vi "ReleaseAllQueues.vi"(8 "error in (no error)":errorcluster, 11 "Message Queues":T1) -> (0 "error out":errorcluster)   [LabVIEW 2018]
uses:
  Message Queue/All Message Queues.ctl
  Message Queue/Message Cluster.ctl
  Controls/Data Queue.ctl
  Controls/Acquired Data.ctl
  Controls/Data Notifier.ctl
  Message Queue/Message Queue.lvlib
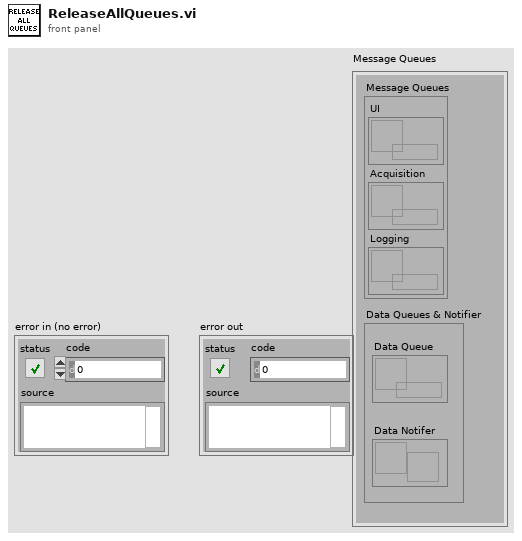
[diagram p1: front panel]
types:
  T1 = typedef "Message Queue.lvlib/All Message Queues.ctl" = cluster{"Message Queues":cluster{"UI":refnum<queue>, "Acquisition":refnum<queue>, "Logging":refnum<queue>}, "Data Queues & Notifier":cluster{"Data Queue":T2, "Data Notifer":T3}}
  T2 = typedef "Data Queue.ctl" = refnum<queue>
  T3 = typedef "Data Notifier.ctl" = refnum<notifier>
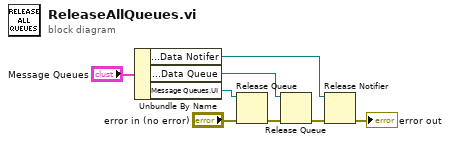
[diagram p0: block diagram]
diagram:
  n1 = Unbundle By Name("Message Queues") -> ("Data Queues & Notifier.Data Notifer"=w3:T3, "Data Queues & Notifier.Data Queue"=w2:T2, "Message Queues.UI"=w1:refnum<queue>)
  n2 = Release Queue(queue=w1, error in (no error)="error in (no error)") -> (error out=w6:errorcluster)  [unwired: 1 in, 2 out]
  n3 = Release Queue(queue=w2, error in (no error)=w6) -> (error out=w7:errorcluster)  [unwired: 1 in, 2 out]
  n4 = Release Notifier(notifier=w3, error in (no error)=w7) -> (error out=→"error out":errorcluster)  [unwired: 1 in, 2 out]
